vi "Up_Hisgram.vi"(7 "Color Mode":u16(ring) items=["RGB", "HSL", "HSV", "HSI"], 8 "error in (no error)":errorcluster, 10 "ROI Descriptor":T2 {"Contours"."Type" items=["No Selection", "Point", "Line", "Rectangle", "Oval", "Polygon", "Free", "Annulus", "Unused2", "Unused3", "Broken Line", "Free Hand Line", "Rotated Rectangle"]}, 11 "Image In":T3) -> (0 "error out":errorcluster, 1 "Histograms":u32[][](array[numeric]), 2 "Statistics":T1 {"Standard  Variation" format="%.2f"; "Mean Value" format="%.2f"; "Maximal Value" format="%.2f"; "Minimal Value" format="%.2f"}, 3 "Image Out":T3)   [LabVIEW 2019]
uses:
  <vilib>/vision/Image Controls.llb/IMAQ Image.ctl
  <vilib>/vision/NI_Vision_Development_Module.lvlib
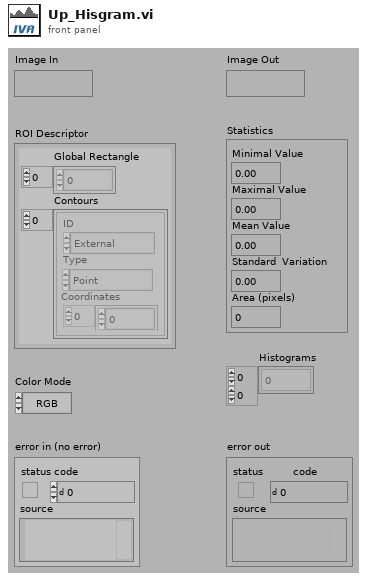
[diagram p1: front panel]
types:
  T1 = cluster{"Minimal Value":sgl, "Maximal Value":sgl, "Mean Value":sgl, "Standard  Variation":sgl, "Area (pixels)":i32}
  T2 = cluster{"Global Rectangle":i32[], "Contours":cluster{"ID":enum32{"External", "Internal"}, "Type":u32, "Coordinates":i32[]}[]}
  T3 = typedef "IMAQ Image.ctl" = refnum<image>
  T4 = cluster{"histogram":u32[], "Minimal Value":sgl, "Maximal Value":sgl, "Starting Value":sgl, "Interval Width":sgl, "Mean Value":sgl, "Standard  Variation":sgl, "Area (pixels)":i32}
  T5 = typedef "Image Type" = u32
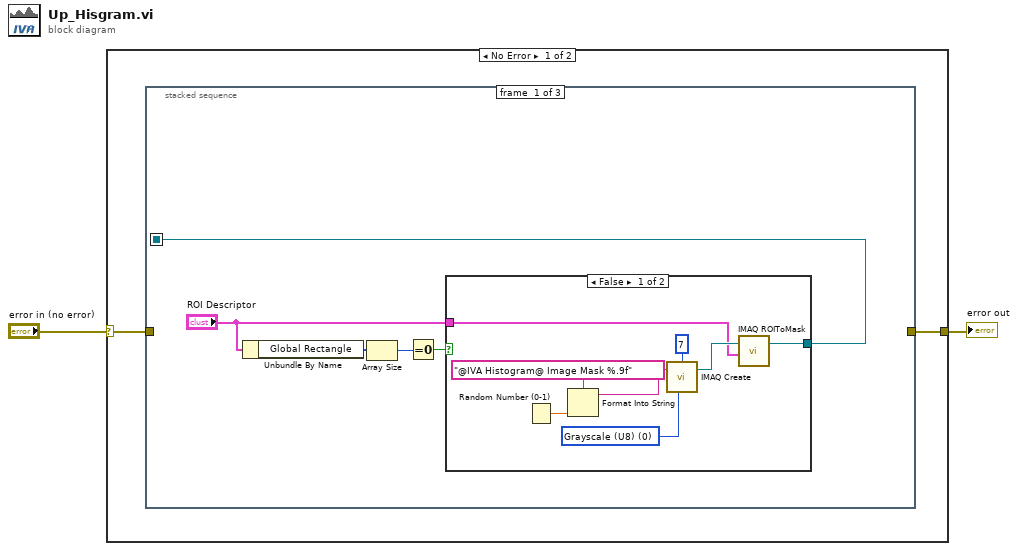
[diagram p0: block diagram]
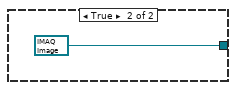
[diagram p2: hidden frame]
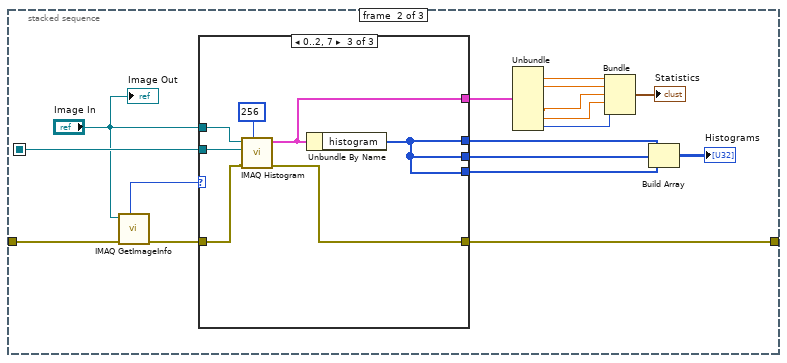
[diagram p3: hidden frame]
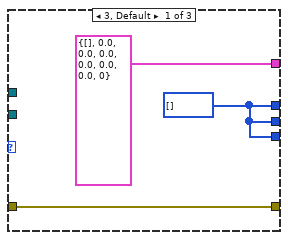
[diagram p4: hidden frame]
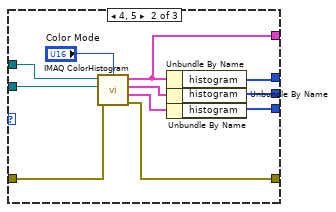
[diagram p5: hidden frame]
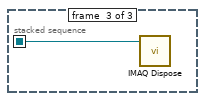
[diagram p6: hidden frame]
diagram:
  n1 = case shown="No Error" "error in (no error)" {
    selector: "error in (no error)" -> [w4 w58]
    tunnel: [w3 w58] -> w2
    frame No Error {
      n2 = stacked-sequence {
        seq-local: [w9 _ _] -> [_ w35 w57]
        tunnel: w4 -> [_ w34 _]
        tunnel: [_ w30 _] -> w3
        frame #0 {
          n3 = Unbundle By Name("ROI Descriptor") -> ("Global Rectangle"=w7:i32[])
          n4 = Array Size(array=w7) -> (size(s)=w6:i32)
          n5 = Equal To 0?(x=w6) -> (x = 0?=w5:bool)
          n6 = case shown="False" w5 {
            tunnel: "ROI Descriptor" -> [w16 _]
            tunnel: [w13 T3 refnum ("Image Out")] -> w9
            frame False {
              w14 = T5 0 items=["Grayscale (U8)", "Grayscale (I16)", "Grayscale (SGL)", "Complex (CSG)", "RGB (U32)", "HSL (U32)", "RGB (U64)", "Grayscale (U16)"] ("Image Type")
              n7 = Random Number (0-1)() -> (number: 0 to 1=w10:dbl)
              n8 = Format Into String(format string="@IVA Histogram@ Image Mask %.9f" ("Image Name"), w10) -> (resulting string=w12:string)  [unwired: 2 in, 1 out]
              n9 = call "IMAQ Create"("Border Size"=7, "Image Name"=w12, "Image Type"=w14) -> ("New Image"=w17:T3)  [unwired: 1 in, 2 out]
              n10 = call "IMAQ ROIToMask"("ROI Descriptor"=w16, "Image"=w17) -> ("Image Out"=w13:T3)  [unwired: 3 in, 3 out]
            }
            frame True {
            }
          }
        }
        frame #1 {
          n11 = call "IMAQ GetImageInfo"("error in (no error)"=w34, "Image"="Image In") -> ("error out"=w33:errorcluster, "Image Type"=w32:T5)  [unwired: 8 out]
          n12 = case shown="0..2, 7" w32 {
            tunnel: w35 -> [_ w49 w56]
            tunnel: "Image In" -> [_ w48 w55]
            tunnel: w33 -> [w37 w46 w54]
            tunnel: [w36 w42 w51] -> w22
            tunnel: [w37 w43 w52] -> w30
            tunnel: [w36 w41 w51] -> w21
            tunnel: [w36 w40 w51] -> w20
            tunnel: [T4 {"histogram"=[], "Minimal Value"=0.0, "Maximal Value"=0.0, "Starting Value"=0.0, "Interval Width"=0.0, "Mean Value"=0.0, "Standard  Variation"=0.0, "Area (pixels)"=0} w39 w50] -> w29
            frame 3, Default {
              w36 = u32[] [] ("histogram")
            }
            frame 4, 5 {
              n13 = call "IMAQ ColorHistogram"("Color Mode"="Color Mode", "Image Src"=w48, "Image Mask"=w49, "error in (no error)"=w46) -> ("Red or Hue or X or L* Histogram Report"=w39:T4, "Green or Sat or Y or a* Histogram Report"=w45:T4, "Blue or Luma or Val or Inten or Z or b* Histogram Report"=w44:T4, "error out"=w43:errorcluster)  [unwired: 2 in]
              n14 = Unbundle By Name(w39) -> ("histogram"=w42:u32[])
              n15 = Unbundle By Name(w45) -> ("histogram"=w41:u32[])
              n16 = Unbundle By Name(w44) -> ("histogram"=w40:u32[])
            }
            frame 0..2, 7 {
              n17 = call "IMAQ Histogram"("Number of Classes"=256, "error in (no error)"=w54, "Image Mask"=w56, "Image"=w55) -> ("error out"=w52:errorcluster, "Histogram Report"=w50:T4)  [unwired: 1 in, 5 out]
              n18 = Unbundle By Name(w50) -> ("histogram"=w51:u32[])
            }
          }
          n19 = Unbundle(w29) -> ("Minimal Value"=w28:sgl, "Maximal Value"=w27:sgl, "Mean Value"=w26:sgl, "Standard  Variation"=w25:sgl, "Area (pixels)"=w24:i32)  [unwired: 3 out]
          n20 = Bundle("Minimal Value"=w28, "Maximal Value"=w27, "Mean Value"=w26, "Standard  Variation"=w25, "Area (pixels)"=w24) -> (→"Statistics":T1)  [unwired: 1 out]
          n21 = Build Array(w22, w21, w20) -> (→"Histograms":u32[][])
          "Image Out" <- "Image In"
        }
        frame #2 {
          n22 = call "IMAQ Dispose"("Image"=w57) -> ()  [unwired: 2 in, 4 out]
        }
      }
    }
    frame Error {
    }
  }
  "error out" <- w2
